vi "Write Multiple Coils.vi"(8 "error in (no error)":errorcluster, 9 "coils":bool[](array[boolean]), 10 "starting address":u16, 11 "device data model in":refnum<class "Standard Data Model.lvclass">) -> (0 "error out":errorcluster, 3 "device data model out":refnum<class "Standard Data Model.lvclass">)   [LabVIEW 2017, in "SubVIs.lvlib" / "Standard Data Model.lvclass"]
doc: "Writes the values of multiple coils in series, starting at address M."
uses:
  <vilib>/Modbus/subvis/Data and Functions/Standard Data Model/Standard Data Model.lvclass
  <vilib>/Modbus/subvis/Data and Functions/Standard Data Model/Standard Data Model.lvclass/Standard Data Model.ctl
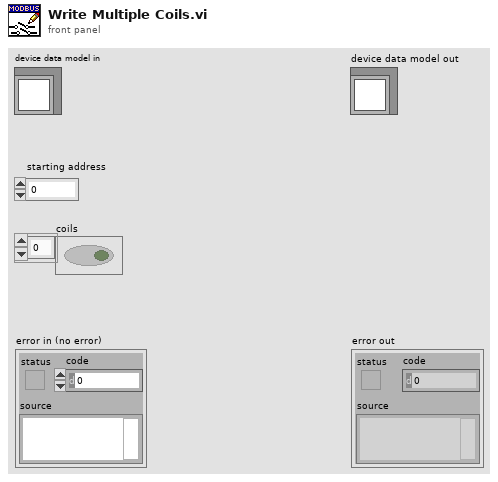
[diagram p1: front panel]
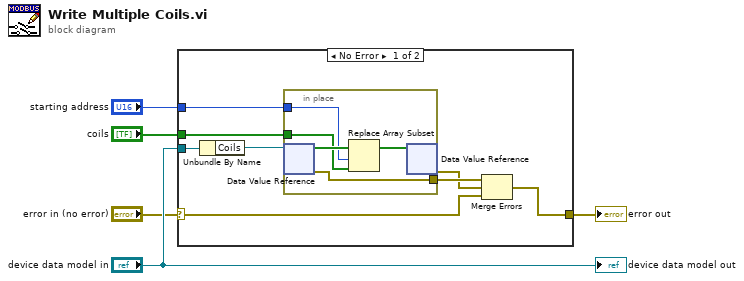
[diagram p0: block diagram]
diagram:
  n1 = case shown="No Error" "error in (no error)" {
    selector: "error in (no error)" -> [w6 w19]
    tunnel: "device data model in" -> [w13 _]
    tunnel: [w12 w19] -> w4
    tunnel: "starting address" -> [w10 _]
    tunnel: "coils" -> [w9 _]
    frame No Error {
      n2 = Unbundle By Name(w13) -> ("Coils"=w11:refnum<data-value>)
      n3 = in-place {
        in-place-border: w10 -> [w16]
        in-place-border: w9 -> [w15]
        in-place-border: [w14] -> w8
        n4 = in-place-dvr #1(w11) -> (w18:bool[], w14:errorcluster)
        n5 = Replace Array Subset(array=w18, new element=w15, index=w16) -> (w17:bool[])
        n6 = in-place-dvr #1(w17) -> (w7:errorcluster)  [unwired: 1 out]
      }
      n7 = Merge Errors(w8, w7, w6) -> (w12:errorcluster)
    }
    frame Error {
    }
  }
  "error out" <- w4
  "device data model out" <- "device data model in"
